vi "Read Exception Status Request.vi"(8 "error in (no error)":errorcluster) -> (0 "error out":errorcluster, 2 "Modbus data unit out":refnum<class "Modbus Data Unit (PDU).lvclass">)   [LabVIEW 2020, in "SubVIs.lvlib" / "Master Function Definition.lvlib"]
doc: "This VI creates the modbus data unit for a read exception status request."
uses:
  <vilib>/Modbus/subvis/Data and Functions/Master Function Definition/Master Function Definition.lvlib
  <vilib>/Modbus/subvis/Modbus Data Unit (PDU)/Modbus Data Unit (PDU).lvclass
  <vilib>/Modbus/subvis/Modbus Data Unit (PDU)/Modbus Data Unit (PDU).lvclass/Modbus Data Unit (PDU).ctl
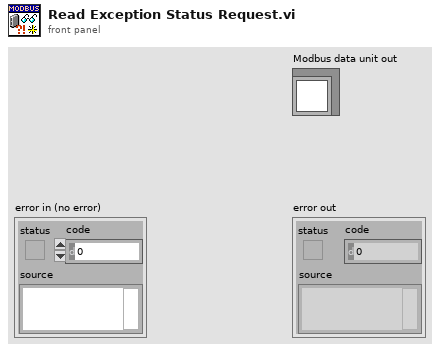
[diagram p1: front panel]
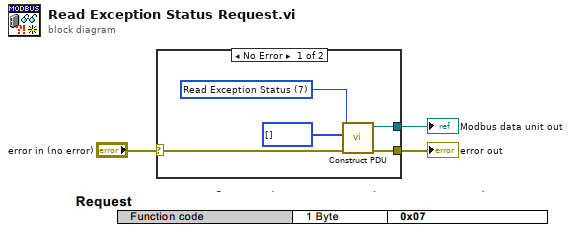
[diagram p0: block diagram]
diagram:
  n1 = case shown="No Error" "error in (no error)" {
    selector: "error in (no error)" -> [w4 w9]
    tunnel: [w8 w9] -> w3
    tunnel: [w7 _] -> w2
    frame No Error {
      w6 = u8 7 items=["Read Discrete Inputs"=2, "Read Coils"=1, "Write Single Coil"=5, "Write Multiple Coils"=15, "Read Input Register"=4, "Read Holding Registers"=3, "Write Single Register"=6, "Write Multiple Registers"=16, "Read/Write Multiple Registers"=23, "Mask Write Register"=22, "Read FIFO Queue"=24, "Read File Record"=20, "Write File Record"=21, "Read Exception Status"=7, "Diagnostic"=8, "Get Com Event Counter"=11, "Get Com Event Log"=12, "Report Slave ID"=17, "Read Device Identification"=43] ("Function")
      n2 = call <vilib>:"Construct PDU.vi"("error in (no error)"=w4, "data"=u8[] [] ("Data"), "function"=w6) -> ("error out"=w8:errorcluster, "Modbus data unit out"=w7:refnum<class "Modbus Data Unit (PDU).lvclass">)  [unwired: 7 in]
    }
    frame Error {
    }
  }
  "error out" <- w3
  "Modbus data unit out" <- w2
